vi "Add Position Measurement Channels.vi"(8 "error in (no error)":errorcluster, 9 "Position Measurement":T1[](array[typedef]) {"ZIndexMode" items=["AHighBHigh"=10040, "AHighBLow"=10041, "ALowBHigh"=10042, "ALowBLow"=10043]; "Decoding" items=["Decoding1X"=10090, "Decoding2X"=10091, "Decoding4X"=10092, "DecodingPulseCounting"=10313]}, 11 "DAQ Ref":refnum<k24>) -> (0 "error out":errorcluster, 3 "DAQ Ref":refnum<k24>)   [LabVIEW 2019, in "Simple SysDef API.lvlib"]
uses:
  <userlib>/SimpleSysDef/Simple SysDef API.lvlib
  NationalInstruments.VeriStand.SystemDefinitionAPI
  <userlib>/SimpleSysDef/_SubVIs/Add Position Measurement Channels_Settings.ctl
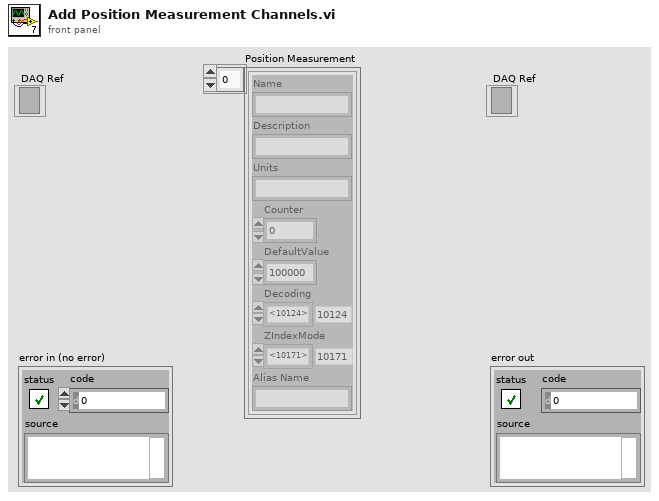
[diagram p1: front panel]
types:
  T1 = typedef "Simple SysDef API.lvlib/Add Position Measurement Channels_Settings.ctl" = cluster{"Name":string, "Description":string, "Units":string, "Counter":u32, "DefaultValue":dbl, "Decoding":i32, "ZIndexMode":i32, "Alias Name":string}
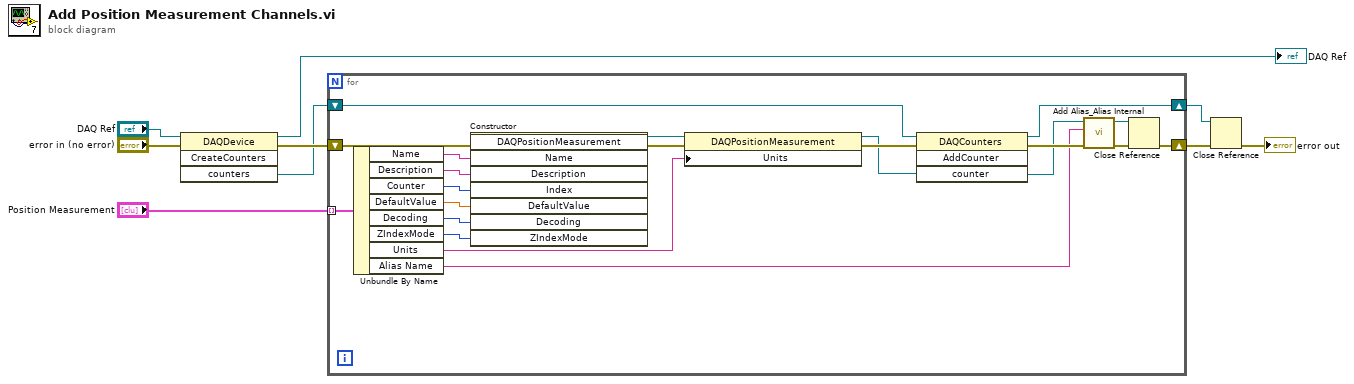
[diagram p0: block diagram]
diagram:
  n1 = invoke class="DAQDevice" method="CreateCounters"(reference="DAQ Ref", error in="error in (no error)") -> (reference out=→"DAQ Ref":refnum<k24>, error out=w4:errorcluster, "counters"=w3:refnum<k24>)  [unwired: 2 in, 1 out]
  n2 = for {
    shift-right: [w27] -> w6
    shift-left: w4 -> [w28]
    shift-right: [w26] -> w7
    shift-left: w3 -> [w29]
    tunnel: "Position Measurement" -> [w22] mode=indexing
    n3 = Unbundle By Name(w22) -> ("Name"=w21:string, "Description"=w20:string, "Counter"=w19:u32, "DefaultValue"=w18:dbl, "Decoding"=w16:i32, "ZIndexMode"=w15:i32, "Units"=w17:string, "Alias Name"=w10:string)
    n4 = constructor class="DAQPositionMeasurement"(error in=w28, "Name"=w21, "Description"=w20, "Index"=w19, "DefaultValue"=w18, "Decoding"=w16, "ZIndexMode"=w15) -> (reference out=w25:refnum<k24>, error out=w24:errorcluster)  [unwired: 2 in, 7 out]
    n5 = property class="DAQPositionMeasurement"(reference=w25, error in=w24, "Units"=w17) -> (reference out=w13:refnum<k24>, error out=w23:errorcluster)
    n6 = invoke class="DAQCounters" method="AddCounter"(reference=w29, error in=w23, "counter"=w13) -> (reference out=w26:refnum<k24>, error out=w14:errorcluster)  [unwired: 1 in, 2 out]
    n7 = call <userlib>:"Add Alias_Alias Internal.vi"("error in (no error)"=w14, "Name"=w10, "Base Node"=w13) -> ("error out"=w11:errorcluster, "Base Node out"=w12:refnum<k24>)  [unwired: 7 in]
    n8 = Close Reference(reference=w12, error in (no error)=w11) -> (error out=w27:errorcluster)
  }
  n9 = Close Reference(reference=w7, error in (no error)=w6) -> (error out=→"error out":errorcluster)
